vi "Get Desired File Extension.vi"(1 "Selected Template VI or CTL name (including file extension)":string) -> (0 "Desired File Extension":T1)   [LabVIEW 2022 SP3]
doc: "This VI decides whether the appropriate file extension for the file about to be created is \".vi\" or \".ctl\".\nIf the user selected a VI or VIT template file, then the new file will be \".vi\".\nIf the user selected a CTT or CTT template file, then the new file will be \".ctl\"."
uses:
  Output File Extension (enum).ctl
panel:
  # "Development\nControls or indicators that are useful for development or testing, but which are not outputs of the VI."
  # "Input\nInputs to the VI"
  # "Output\nOutputs of the VI"
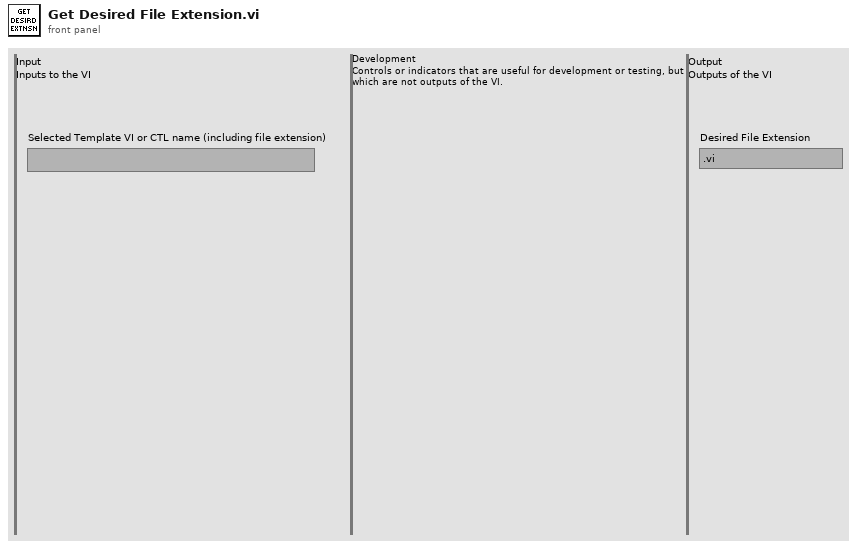
[diagram p1: front panel]
types:
  T1 = typedef "Output File Extension (enum).ctl" = enum16{".vi", ".ctl"}
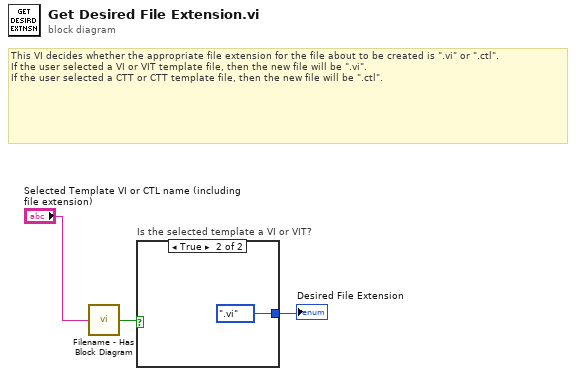
[diagram p0: block diagram]
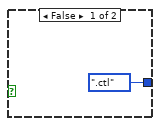
[diagram p2: hidden frame]
diagram:
  # "This VI decides whether the appropriate file extension for the file about to be created is \".vi\" or \".ctl\".\nIf the user selected a VI or VIT template file, then the new file will be \".vi\".\nIf the user selected a CTT or CTT template file, then the new file will be \".ctl\"."
  n1 = call "Filename - Has Block Diagram.vi"("Filename (including file extension)"="Selected Template VI or CTL name (including file extension)") -> ("Has Block Diagram?"=w3:bool)
  n2 = case "Is the selected template a VI or VIT?" shown="True" w3 {
    tunnel: [Output_File_Extension_(enum).".ctl" ("Output File Extension") Output_File_Extension_(enum).".vi" ("Output File Extension")] -> w1
    frame False {
    }
    frame True {
    }
  }
  "Desired File Extension" <- w1
